vi "Sign (Private Key Bytes).vi"(5 "RSASignPadding":T2, 7 "HashingAlgorithm":T1=enum."SHA512", 8 "error in (no error)":errorcluster, 10 "Data in":u8[](array[numeric]), 11 "Private key (bytes)":u8[](array[numeric])) -> (0 "error out":errorcluster, 2 "Signature out":u8[](array[numeric]))   [LabVIEW 2021, in "dotNET Crypto Asymmetric Encryption.lvlib"]
doc: "Generate a signature from the data using the private key."
uses:
  dotNET Crypto Asymmetric Encryption.lvlib
  RSASignaturePadding.ctl
  Utility/HashingAlgorithm.ctl
  System.Core
  Utility/dotNET Crypto Utility.lvlib
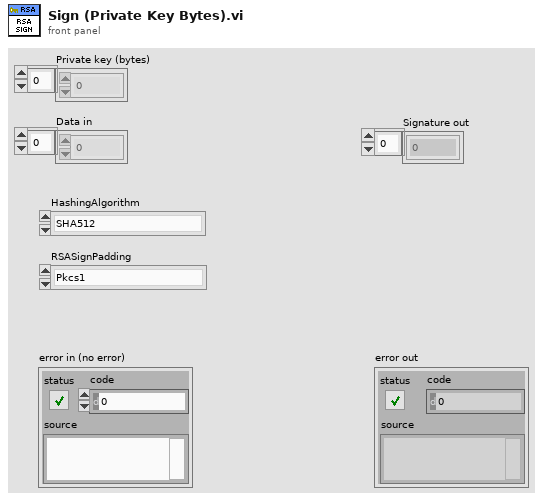
[diagram p1: front panel]
types:
  T1 = typedef "dotNET Crypto Utility.lvlib/HashingAlgorithm.ctl" = enum16{"MD5", "SHA1", "SHA256", "SHA384", "SHA512"}
  T2 = typedef "dotNET Crypto Asymmetric Encryption.lvlib/RSASignaturePadding.ctl" = enum16{"Pkcs1", "Pss"}
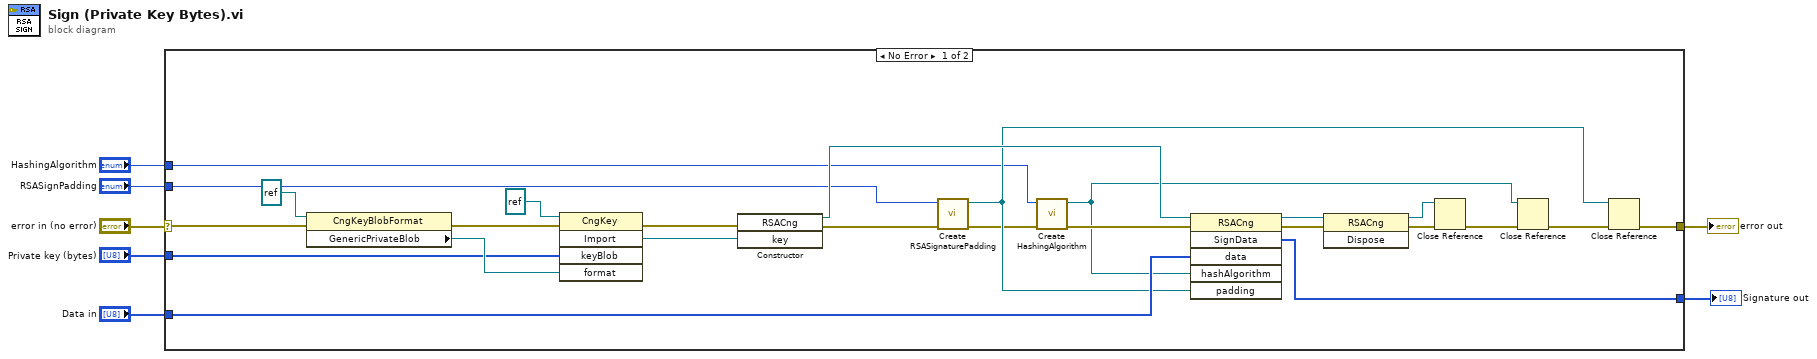
[diagram p0: block diagram]
diagram:
  n1 = case shown="No Error" "error in (no error)" {
    selector: "error in (no error)" -> [w11 w33]
    tunnel: "Data in" -> [w32 _]
    tunnel: [w31 _] -> w6
    tunnel: "RSASignPadding" -> [w23 _]
    tunnel: "HashingAlgorithm" -> [w17 _]
    tunnel: [w16 w33] -> w3
    tunnel: "Private key (bytes)" -> [w8 _]
    frame No Error {
      n2 = property class="CngKeyBlobFormat"(reference=refnum<k24> refnum ("format"), error in=w11) -> (error out=w13:errorcluster, "GenericPrivateBlob"=w12:refnum<k24>)  [unwired: 1 out]
      n3 = invoke class="CngKey" method="Import"(reference=refnum<k24> refnum, error in=w13, "keyBlob"=w8, "format"=w12) -> (error out=w10:errorcluster, "Import"=w9:refnum<k24>)  [unwired: 1 in, 3 out]
      n4 = constructor class="RSACng"(error in=w10, "key"=w9) -> (reference out=w25:refnum<k24>, error out=w26:errorcluster)  [unwired: 2 in, 2 out]
      n5 = call "Create RSASignaturePadding.vi"("error in (no error)"=w26, "RSASignaturePadding"=w23) -> ("error out"=w22:errorcluster, "RSASignaturePadding out"=w24:refnum<k24>)  [unwired: 8 in]
      n6 = call "Create HashingAlgorithm.vi"("error in (no error)"=w22, "HashingAlgorithm"=w17) -> ("error out"=w21:errorcluster, "Hashing Algorithm"=w18:refnum<k24>)  [unwired: 8 in]
      n7 = invoke class="RSACng" method="SignData"(reference=w25, error in=w21, "data"=w32, "hashAlgorithm"=w18, "padding"=w24) -> (reference out=w29:refnum<k24>, error out=w30:errorcluster, "SignData"=w31:u8[])  [unwired: 1 in, 3 out]
      n8 = invoke class="RSACng" method="Dispose"(reference=w29, error in=w30) -> (reference out=w28:refnum<k24>, error out=w27:errorcluster)  [unwired: 1 in, 1 out]
      n9 = Close Reference(reference=w28, error in (no error)=w27) -> (error out=w20:errorcluster)
      n10 = Close Reference(reference=w18, error in (no error)=w20) -> (error out=w19:errorcluster)
      n11 = Close Reference(reference=w24, error in (no error)=w19) -> (error out=w16:errorcluster)
    }
    frame Error {
    }
  }
  "error out" <- w3
  "Signature out" <- w6
